vi "Prober_ChuckUpDown.vi"(8 "error in (no error)":errorcluster, 10 "Direction":enum16{"up", "down"}(ring), 11 "TeslaVeloxProbeStation in":refnum<class "TeslaVeloxProbeStation.lvclass">) -> (0 "error out":errorcluster, 2 "Chuck at CONTACT?":bool=TRUE, 3 "TeslaVeloxProbeStation out":refnum<class "TeslaVeloxProbeStation.lvclass">)   [LabVIEW 2018, in "TeslaVeloxProbeStation.lvclass"]
uses:
  TeslaVeloxProbeStation.lvclass
  ProbeStationControl.lvclass
  Desktop/Kvasnicka/test_labview_library/Integration_toolkit_library/CascadeProbestation.lvlib
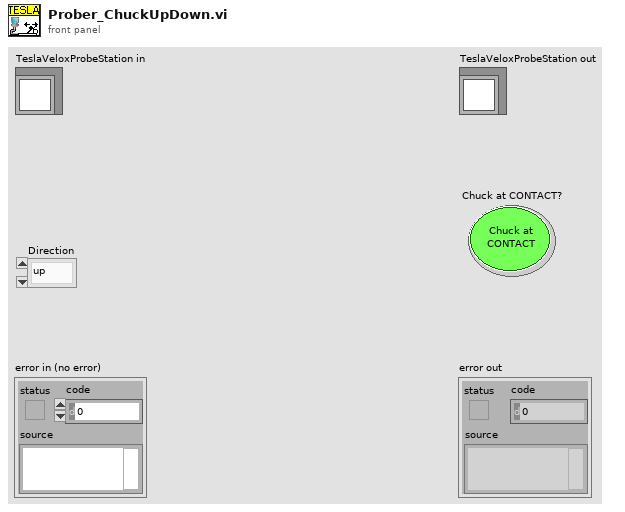
[diagram p1: front panel]
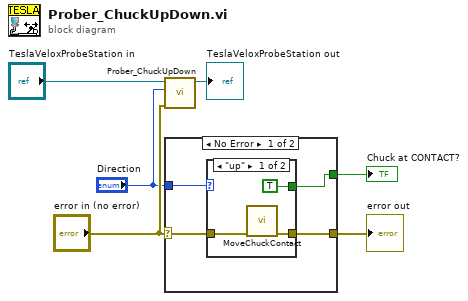
[diagram p0: block diagram]
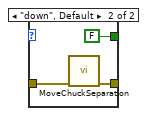
[diagram p2: hidden frame]
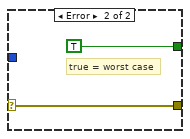
[diagram p3: hidden frame]
diagram:
  n1 = call-parent "Prober_ChuckUpDown.vi"("error in (no error)"="error in (no error)", "Direction"="Direction", "ProbeStationControl in"="TeslaVeloxProbeStation in") -> ("ProbeStationControl out"=→"TeslaVeloxProbeStation out":refnum<class "TeslaVeloxProbeStation.lvclass">)  [unwired: 6 in, 2 out]
  n2 = case shown="No Error" "error in (no error)" {
    selector: "error in (no error)" -> [w9 w18]
    tunnel: "Direction" -> [w10 _]
    tunnel: [w8 w18] -> w2
    tunnel: [w7 TRUE ("Chuck at CONTACT?")] -> w1
    frame No Error {
      n3 = case shown="\"up\"" w10 {
        tunnel: w9 -> [w13 w16]
        tunnel: [w12 w15] -> w8
        tunnel: [TRUE ("Chuck at CONTACT?") FALSE ("Chuck at CONTACT?")] -> w7
        frame "up" {
          n4 = call "MoveChuckContact.vi"("Error In"=w13) -> ("Error Out"=w12:errorcluster)  [unwired: 9 in, 1 out]
        }
        frame "down", Default {
          n5 = call "MoveChuckSeparation.vi"("Error In"=w16) -> ("Error Out"=w15:errorcluster)  [unwired: 9 in, 1 out]
        }
      }
    }
    frame Error {
      # "true = worst case"
    }
  }
  "error out" <- w2
  "Chuck at CONTACT?" <- w1
